vi "U01_6DBQuery.vi"() -> ()   [LabVIEW 2015]
uses:
  <vilib>/addons/database/Connection.llb/DB Tools Open Connec (Path).vi
  <vilib>/addons/database/NI_Database_API.lvlib
  <vilib>/addons/database/_DB Variant To Data/Database Variant To Data.xnode
panel:
  out "data 2":variant[][](array[variant])
  out "error out":errorcluster
  out "data":variant
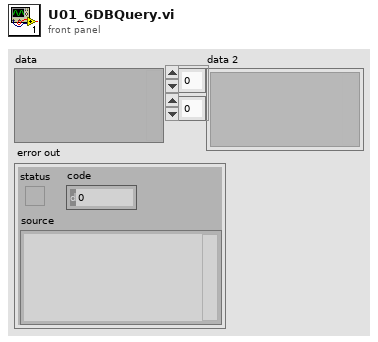
[diagram p1: front panel]
types:
  T1 = typedef "NI_Database_API.lvlib/Conn ObjectReference.ctl" = refnum<k1>
  T2 = cluster{"Clave":i32, "Estado":string, "Temperatura":dbl, "Fecha":string}
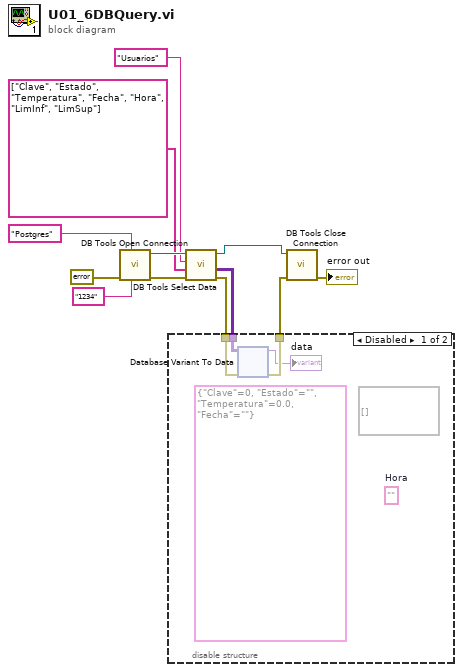
[diagram p0: block diagram]
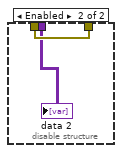
[diagram p2: hidden frame]
diagram:
  n1 = call-poly <vilib>:"DB Tools Open Connection.vi"("password"="1234", "userID"="Postgres", "error in (no error)"=errorcluster {"status"=FALSE, "code"=0, "source"=""}) -> ("error out"=w9:errorcluster, "connection reference"=w10:T1)  [unwired: 5 in]
  n2 = call <vilib>:"DB Tools Select Data.vi"("error in (no error)"=w9, "columns"=string[] ["Clave", "Estado", "Temperatura", "Fecha", "Hora", "LimInf", "LimSup"], "table"="Usuarios", "connection reference"=w10) -> ("error out"=w3:errorcluster, "data"=w4:variant[][], "connection reference out"=w5:T1)  [unwired: 2 in]
  n3 = disable-structure shown="Disabled" {
    disable-tunnel: w4 -> [w16 w52]
    disable-tunnel: w3 -> [w15 w53]
    disable-tunnel: [w14 w53] -> w2
    frame Disabled {
      (unwired) ""  # Hora
      (unwired) T2 {"Clave"=0, "Estado"="", "Temperatura"=0.0, "Fecha"=""}
      (unwired) void[] []
      n4 = xnode "Database Variant To Data"("database variant"=w16, "error in (no error)"=w15) -> ("data"=→"data":variant, "error out"=w14:errorcluster)  [unwired: 1 in]
    }
    frame Enabled {
      "data 2" <- w52
    }
  }
  n5 = call <vilib>:"DB Tools Close Connection.vi"("error in (no error)"=w2, "connection reference"=w5) -> ("error out"=→"error out":errorcluster)  [unwired: 5 in]
